vi "LV SciSDK SPECTRUM RESET.vi"(8 "error in (no error)":errorcluster, 9 "Board Handle In":T1, 10 "Handle In":T2) -> (0 "error out":errorcluster, 1 "Board Handle Out":T1, 2 "Handle Out":T2, 3 "NI Error Code":i32)   [LabVIEW 2021, in "SciSDK_Labview.lvlib"]
uses:
  SciSDK_Labview.lvlib
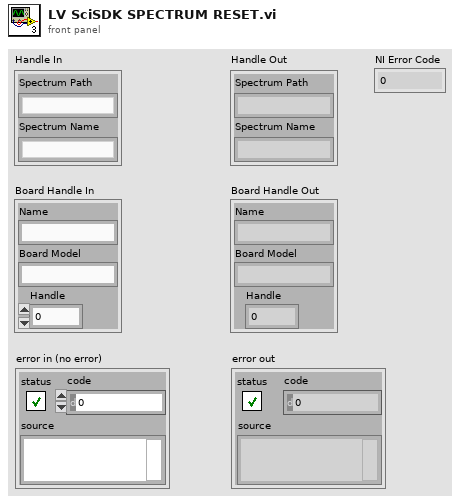
[diagram p1: front panel]
types:
  T1 = cluster{"Name":string, "Board Model":string, "Handle":u64}
  T2 = cluster{"Spectrum Path":string, "Spectrum Name":string}
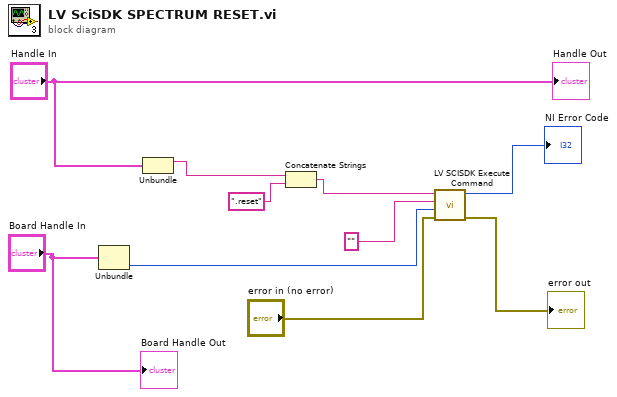
[diagram p0: block diagram]
diagram:
  n1 = Unbundle("Board Handle In") -> ("Handle"=w2:u64)  [unwired: 2 out]
  n2 = Unbundle("Handle In") -> ("Spectrum Path"=w4:string)  [unwired: 1 out]
  n3 = Concatenate Strings(w4, ".reset" ("string")) -> (w9:string)
  n4 = call "LV SCISDK Execute Command.vi"("error in (no error)"="error in (no error)", "handle"=w2, "value"="", "Path"=w9) -> ("error out"=→"error out":errorcluster, "function return"=→"NI Error Code":i32)  [unwired: 5 in, 1 out]
  "Handle Out" <- "Handle In"
  "Board Handle Out" <- "Board Handle In"
